vi "FTW-Ether-CreateListener.vi"(5 "Endpoint Type":T2, 7 "Message Transport Scheme":T1, 11 "error in":errorcluster) -> (4 "FTW-Listener":refnum<class "FTW-Listener.lvclass">, 15 "error out":errorcluster)   [LabVIEW 2013, in "FTW-Ether.lvclass"]
uses:
  FTW-Ether.lvclass
  Listener/FTW-Listener.lvclass
  FTW-Ether-EndpointType.ctl
  FTW-Ether-MessageTransportScheme.ctl
  Listener-TCP/FTW-Listener-TCP.lvclass
  Listener-LVQ/FTW-Listener-LVQ.lvclass
panel:
  # "Inputs"
  # "Outputs"
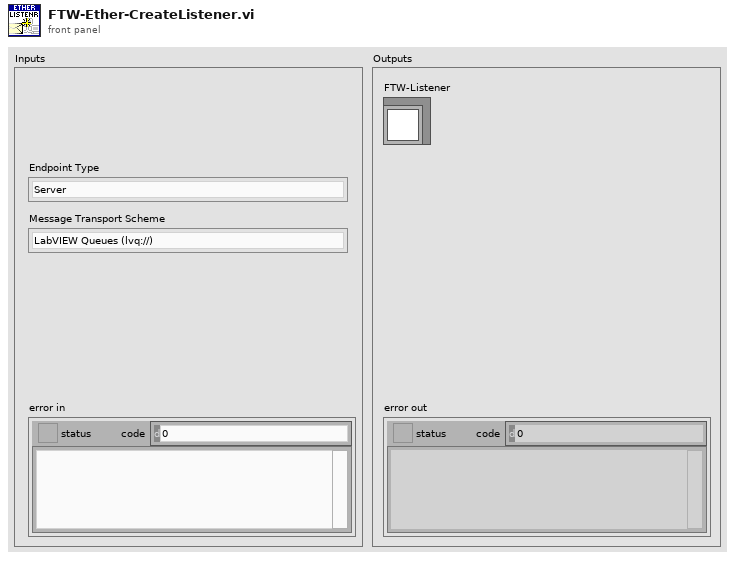
[diagram p1: front panel]
types:
  T1 = typedef "FTW-Ether.lvclass/FTW-Ether-MessageTransportScheme.ctl" = enum16{"LabVIEW Queues (lvq://)", "TCP (tcp://)", "LabVIEW Notifiers (lvn://)", "LabVIEW Network Streams (lvns://)"}
  T2 = typedef "FTW-Ether.lvclass/FTW-Ether-EndpointType.ctl" = enum16{"Server", "Client", "Publisher", "Subscriber"}
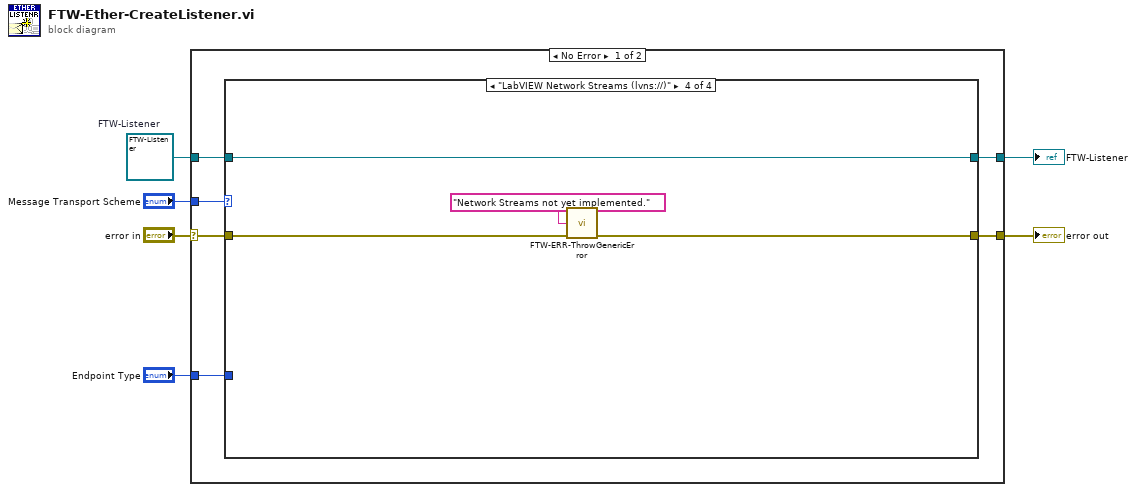
[diagram p0: block diagram]
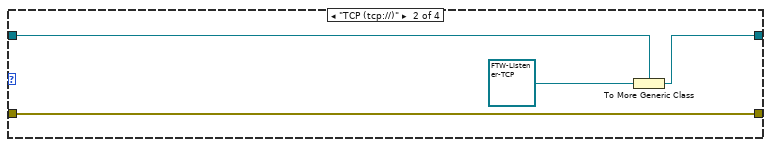
[diagram p3: hidden frame]
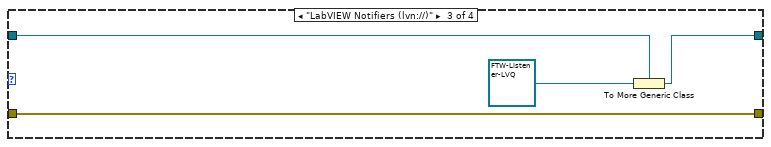
[diagram p4: hidden frame]
diagram:
  w1 = refnum<class "FTW-Listener.lvclass"> refnum  # FTW-Listener
  n1 = case shown="No Error" "error in" {
    selector: "error in" -> [w9 w28]
    tunnel: [w12 w27] -> w6
    tunnel: [w11 w28] -> w5
    tunnel: "Message Transport Scheme" -> [w10 _]
    tunnel: "Endpoint Type" -> [w8 _]
    tunnel: w1 -> [w7 w27]
    frame No Error {
      n2 = case shown="\"LabVIEW Network Streams (lvns://)\"" w10 {
        tunnel: [w14 w16 w20 w23] -> w12
        tunnel: [w13 w18 w22 w24] -> w11
        tunnel: w9 -> [w13 w18 w22 w25]
        tunnel: w8 -> [_ _ _ _]
        tunnel: w7 -> [w14 w17 w21 w23]
        frame "LabVIEW Queues (lvq://)" {
        }
        frame "TCP (tcp://)" {
          n3 = To More Generic Class(target class=w17, reference=refnum<class "FTW-Listener-TCP.lvclass"> refnum ("Featherweight Actor:FTW Endpoint")) -> (generic class reference=w16:refnum<class "FTW-Listener.lvclass">)
        }
        frame "LabVIEW Notifiers (lvn://)" {
          n4 = To More Generic Class(target class=w21, reference=refnum<class "FTW-Listener-LVQ.lvclass"> refnum ("Featherweight Actor:FTW Endpoint")) -> (generic class reference=w20:refnum<class "FTW-Listener.lvclass">)
        }
        frame "LabVIEW Network Streams (lvns://)" {
          n5 = call "FTW-ERR-ThrowGenericError.vi"("Error Message"="Network Streams not yet implemented.", "error in"=w25) -> ("error out"=w24:errorcluster)  [unwired: 13 in]
        }
      }
    }
    frame Error {
    }
  }
  "error out" <- w5
  "FTW-Listener" <- w6
